vi "事件捕捉器.vi"() -> ()   [LabVIEW 2018]
panel:
  out "Other Parameters":sgl[](array[numeric])
  out "Coordinates":i32[](array[numeric])
  out "Tool":i32(ring) items=["Point", "Line", "Rectangle", "Oval", "Polygon", "Freehand Region", "Annulus", "Rotated Rectangle", "Zoom", "Pan", "Broken Line", "Freehand Line"]
  out "Event":i32(ring) items=["No  event", "Click event", "Draw event", "Move event", "Size event", "Scroll event", "Activate event", "Close event", "Double click event"]
  in  "布尔":bool
  in  "路径":path
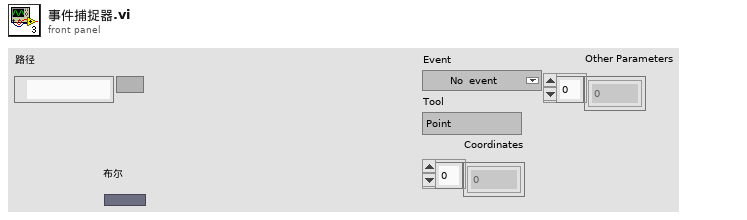
[diagram p1: front panel]
types:
  T1 = typedef "Image Type" = u32
  T2 = typedef "IMAQ Image.ctl" = refnum<image>
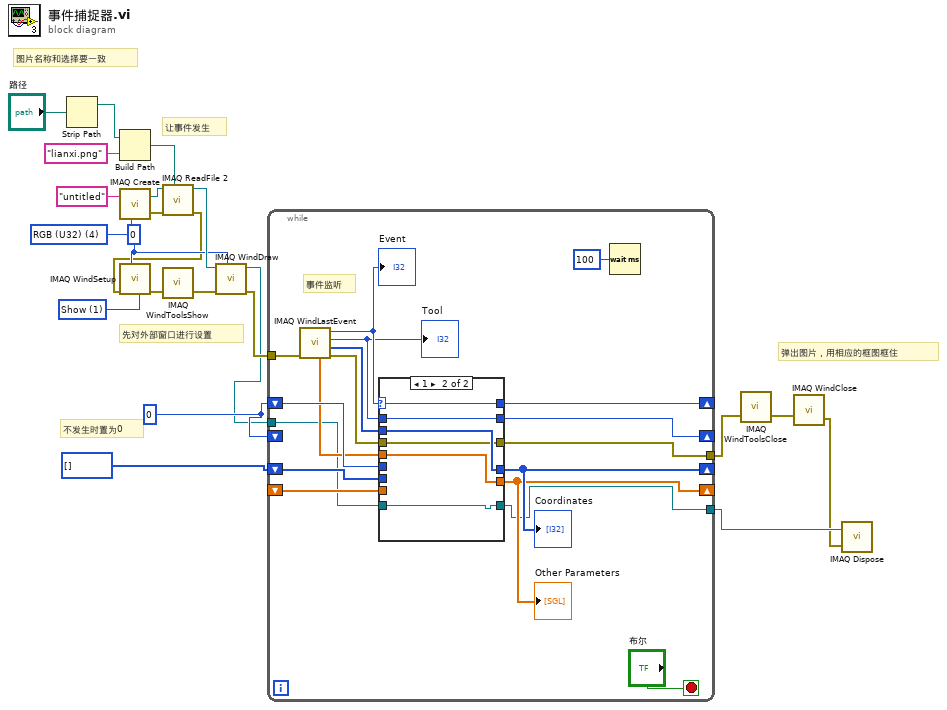
[diagram p0: block diagram]
diagram:
  w8 = 0 ("Event")
  w10 = 1 items=["Hide", "Show", "No change"] ("Scrollbars (No change)")
  w11 = 0 ("Window Number (0...15)")
  w15 = T1 4 items=["Grayscale (U8)", "Grayscale (I16)", "Grayscale (SGL)", "Complex (CSG)", "RGB (U32)", "HSL (U32)", "RGB (U64)", "Grayscale (U16)"] ("Image Type")
  # "图片名称和选择要一致"
  # "弹出图片，用相应的框图框住"
  # "不发生时置为0"
  # "让事件发生"
  # "先对外部窗口进行设置"
  n1 = Strip Path(path="路径") -> (stripped path=w21:path)  [unwired: 1 out]
  n2 = Build Path(base path=w21, name or relative path="lianxi.png" ("名称或相对路径")) -> (appended path=w19:path)
  n3 = call "IMAQ Create"("Image Name"="untitled", "Image Type"=w15) -> ("New Image"=w18:T2, "error out"=w17:errorcluster)  [unwired: 3 in]
  n4 = call "IMAQ ReadFile 2"("File Path"=w19, "error in (no error)"=w17, "Image"=w18) -> ("error out"=w1:errorcluster, "Image Out"=w14:T2)  [unwired: 4 in, 3 out]
  n5 = call "IMAQ WindSetup"("Scrollbars (No change)"=w10, "Window Number (0...15)"=w11, "error in (no error)"=w1) -> ("error out"=w13:errorcluster)  [unwired: 8 in]
  n6 = call "IMAQ WindToolsShow"("error in (no error)"=w13) -> ("error out"=w12:errorcluster)  [unwired: 4 in, 1 out]
  n7 = call "IMAQ WindDraw"("Window Number (0...15)"=w11, "error in (no error)"=w12, "Image"=w14) -> ("error out"=w9:errorcluster, "Image Out (duplicate)"=w4:T2)  [unwired: 7 in]
  n8 = while {
    tunnel: w9 -> [w40]
    shift-right: [w38] -> _
    shift-left: w8 -> [w36]
    shift-right: [w34] -> _
    shift-left: w8 -> [_]
    shift-right: [w32] -> _
    shift-left: i32[] [] ("Coordinates") -> [w31]
    shift-right: [w29] -> _
    shift-left: _ -> [w28]
    tunnel: [w26] -> w5
    tunnel: w4 -> [w25]
    tunnel: [w23] -> w3
    stop <- "布尔" stop-if-true
    # "事件监听"
    n9 = call "IMAQ WindLastEvent"("error in (no error)"=w40) -> ("error out"=w27:errorcluster, "Coordinates"=w33:i32[], "Tool"=w35:i32, "Event"=w37:i32, "Other Parameters"=w30:sgl[])  [unwired: 5 in, 1 out]
    "Event" <- w37
    "Tool" <- w35
    n10 = case shown="1" w37 {
      selector: w37 -> [_ w52]
      tunnel: [w46 w52] -> w38
      tunnel: w36 -> [w46 _]
      tunnel: w35 -> [w44 w51]
      tunnel: [w44 w51] -> w34
      tunnel: w33 -> [_ w50]
      tunnel: [w45 w50] -> w32
      tunnel: w31 -> [w45 _]
      tunnel: w30 -> [_ w49]
      tunnel: [w43 w49] -> w29
      tunnel: w28 -> [w43 _]
      tunnel: w27 -> [w42 w48]
      tunnel: [w42 w48] -> w26
      tunnel: [w41 w47] -> w23
      tunnel: w25 -> [w41 w47]
      frame 0, Default {
      }
      frame 1 {
      }
    }
    "Coordinates" <- w32
    "Other Parameters" <- w29
    n11 = Wait (ms)(milliseconds to wait=u32 100 ("等待时间（毫秒）")) -> ()  [unwired: 1 out]
  }
  n12 = call "IMAQ WindToolsClose"("error in (no error)"=w5) -> ("error out"=w6:errorcluster)  [unwired: 5 in]
  n13 = call "IMAQ WindClose"("error in (no error)"=w6) -> ("error out"=w2:errorcluster)  [unwired: 5 in]
  n14 = call "IMAQ Dispose"("Image"=w3, "error in (no error)"=w2) -> ()  [unwired: 4 in, 1 out]
